vi "PV generator zen42 Laurent V3.vi"(8 "errin":errorcluster, 10 "network":path, 11 "path in":path) -> (0 "sortie d'erreur":errorcluster caption="errout", 2 "network out":path, 3 "tout bon":bool)   [LabVIEW 2017]
uses:
  <vilib>/Utility/config.llb/NI_LVConfig.lvlib
panel:
  out "Array 3":dbl[](array[numeric])
  out "nombre de remplacements":i32
  out "Chaîne":string
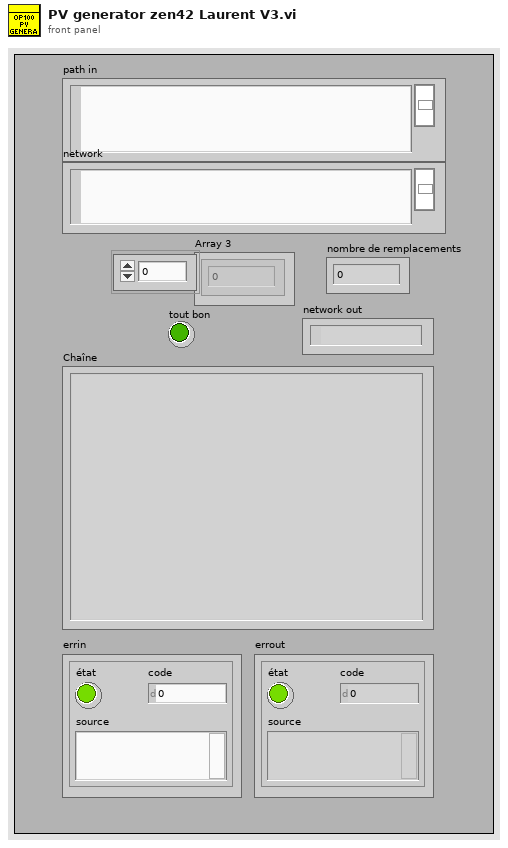
[diagram p1: front panel]
types:
  T1 = enum16{"open", "replace", "create", "open or create", "replace or create", "replace or create with confirmation"}
  T2 = typedef "NI_LVConfig.lvlib/Config Data RefNum.ctl" = refnum<k1>
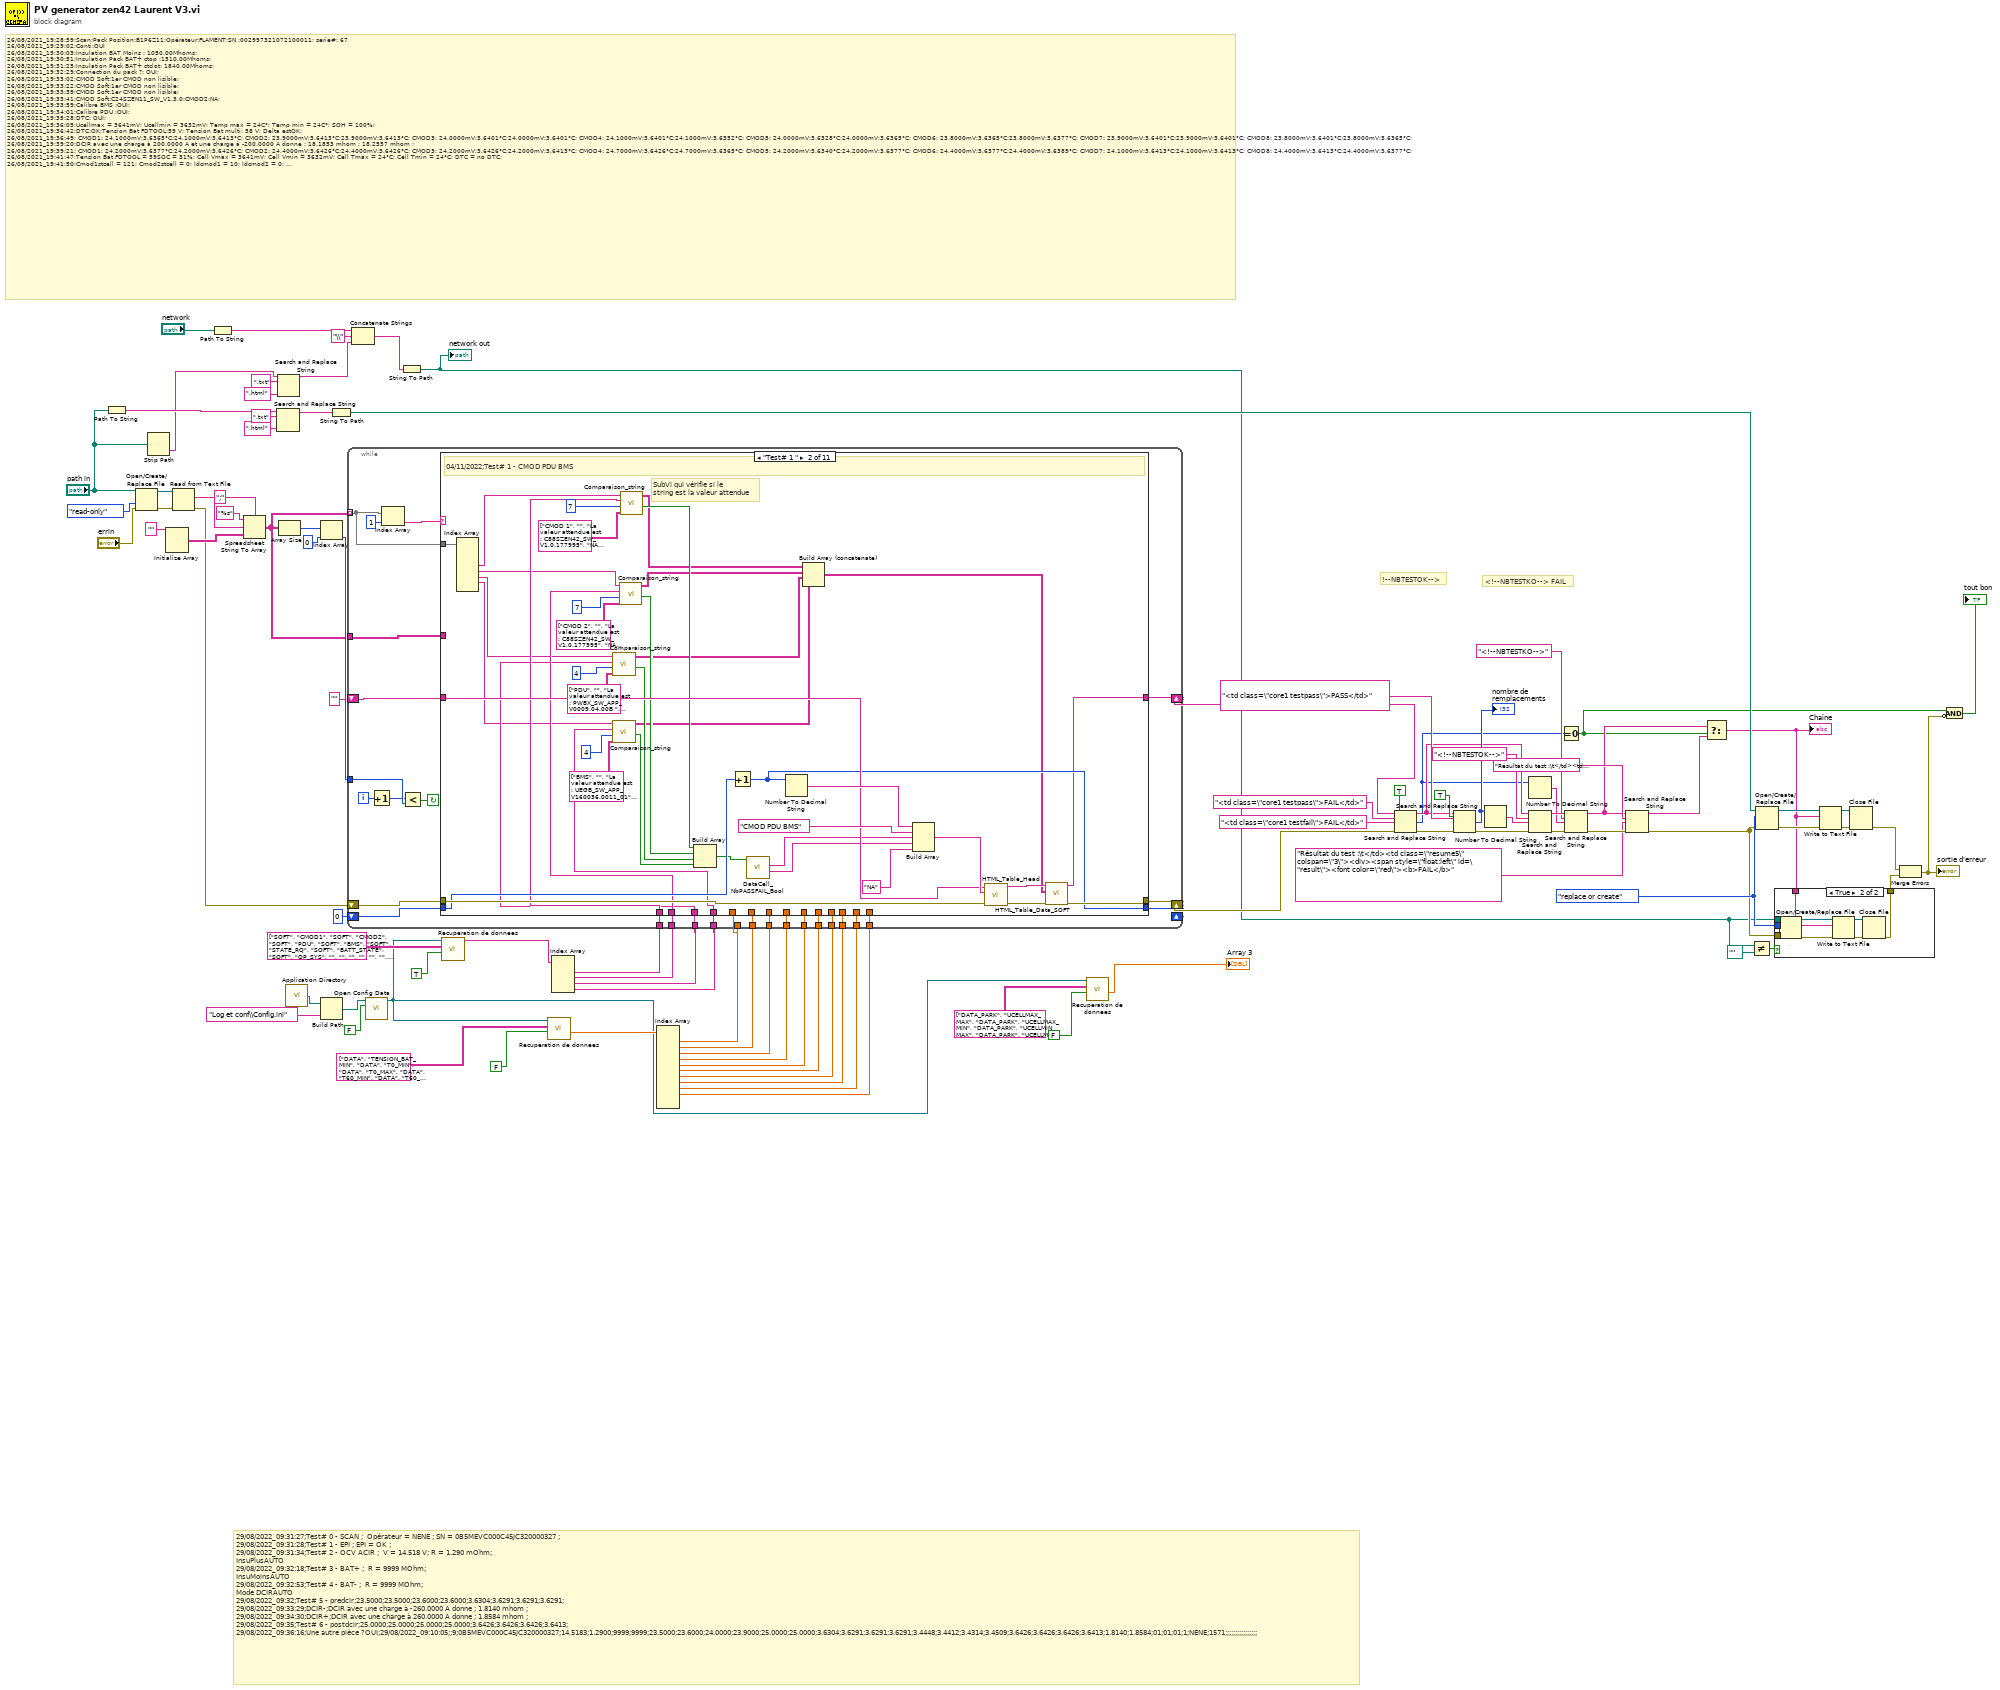
[diagram p0: block diagram]
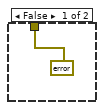
[diagram p2: hidden frame]
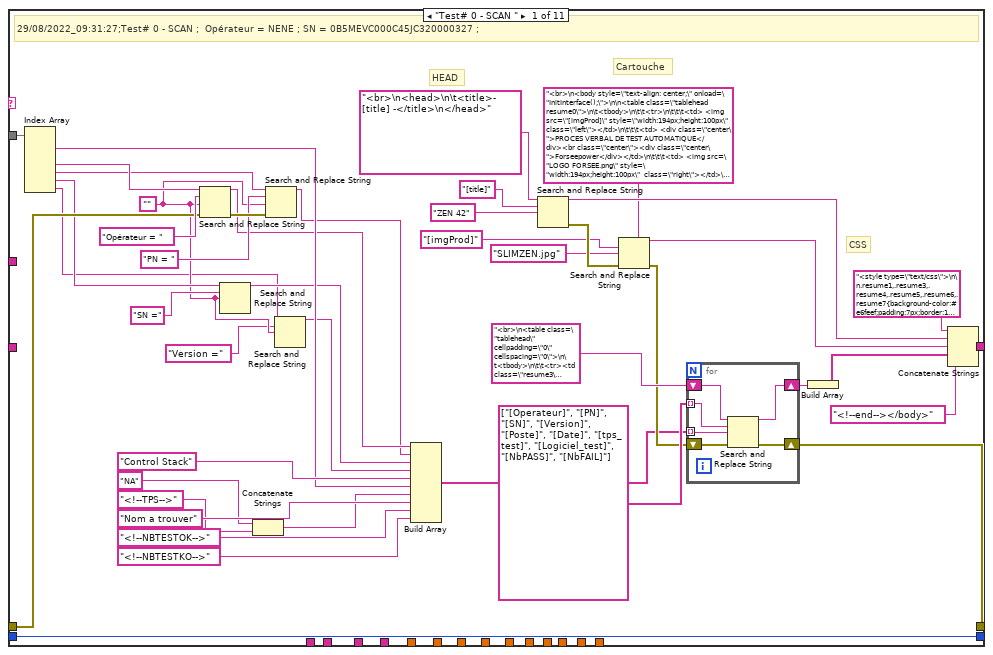
[diagram p3: hidden frame]
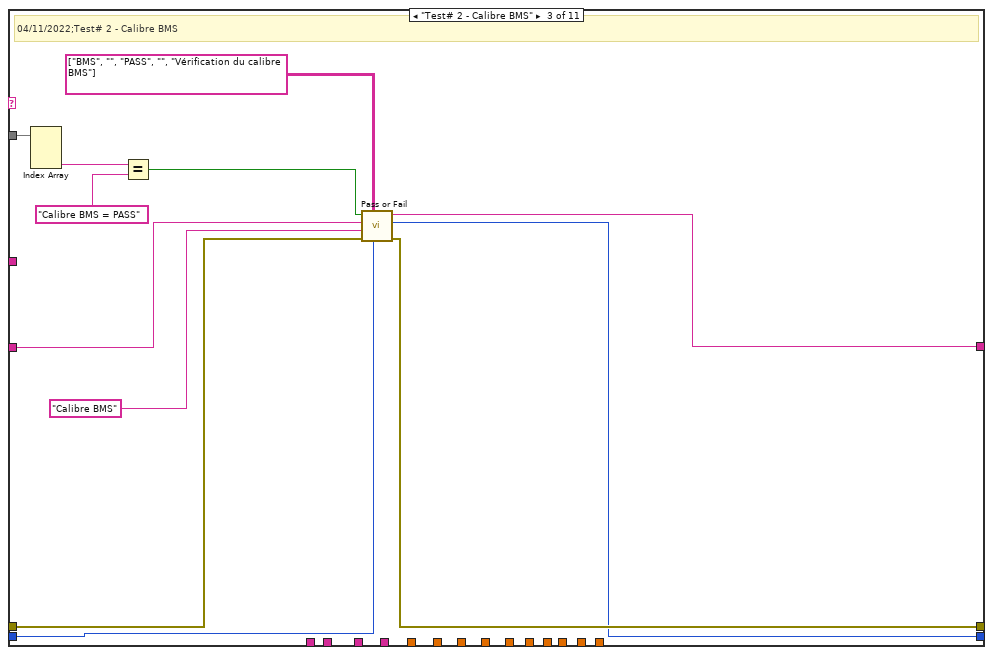
[diagram p4: hidden frame]
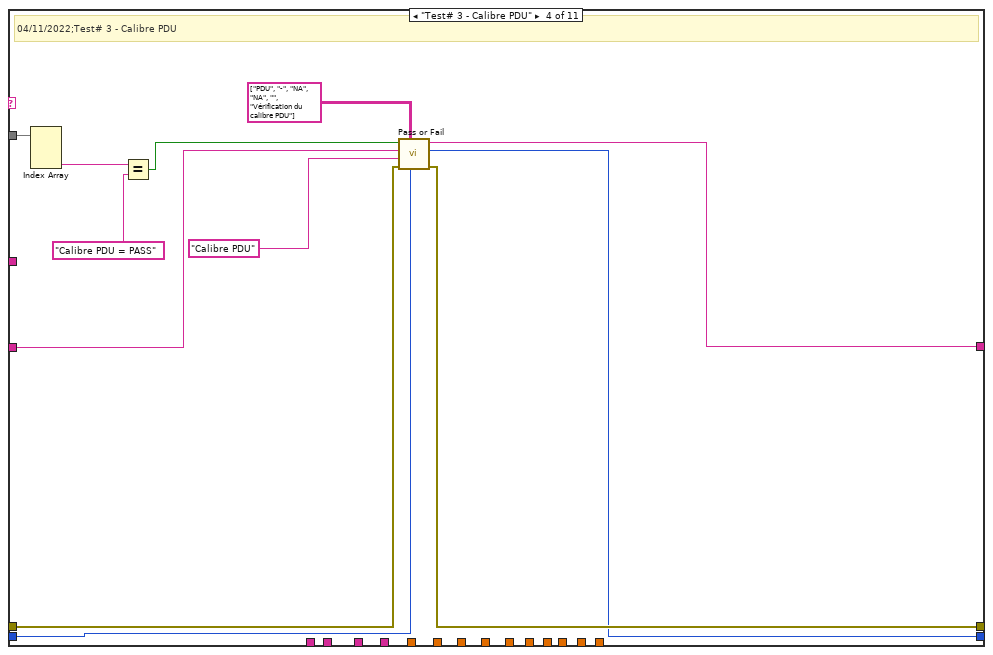
[diagram p5: hidden frame]
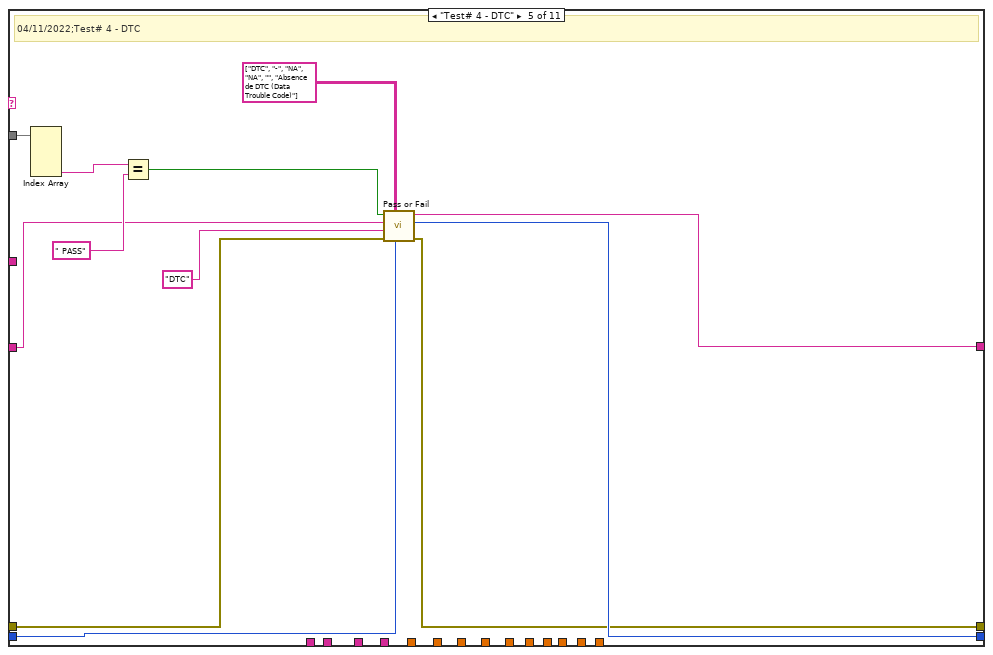
[diagram p6: hidden frame]
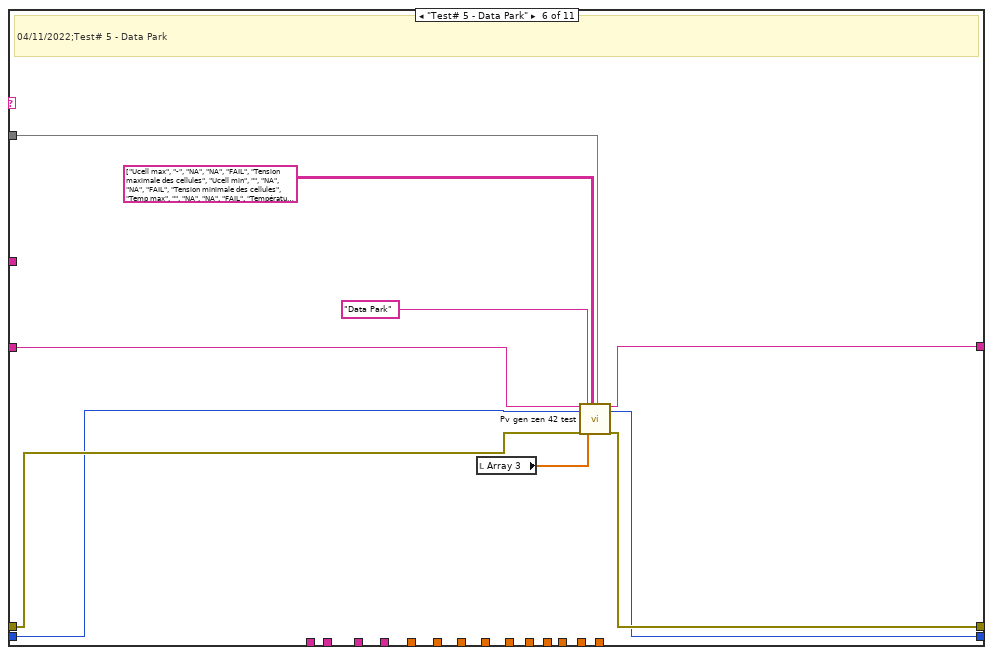
[diagram p7: hidden frame]
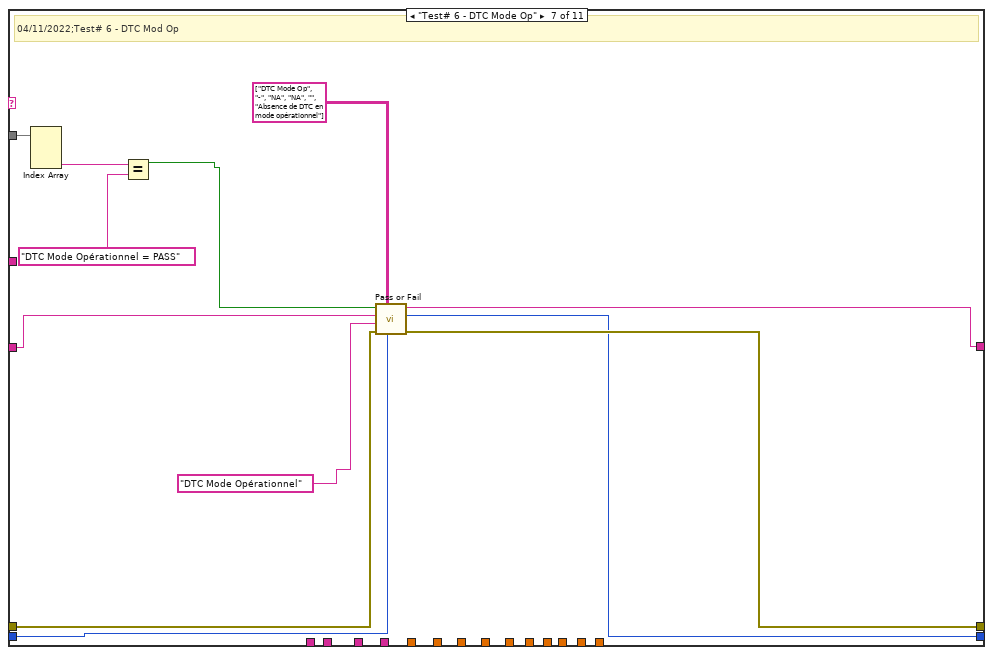
[diagram p8: hidden frame]
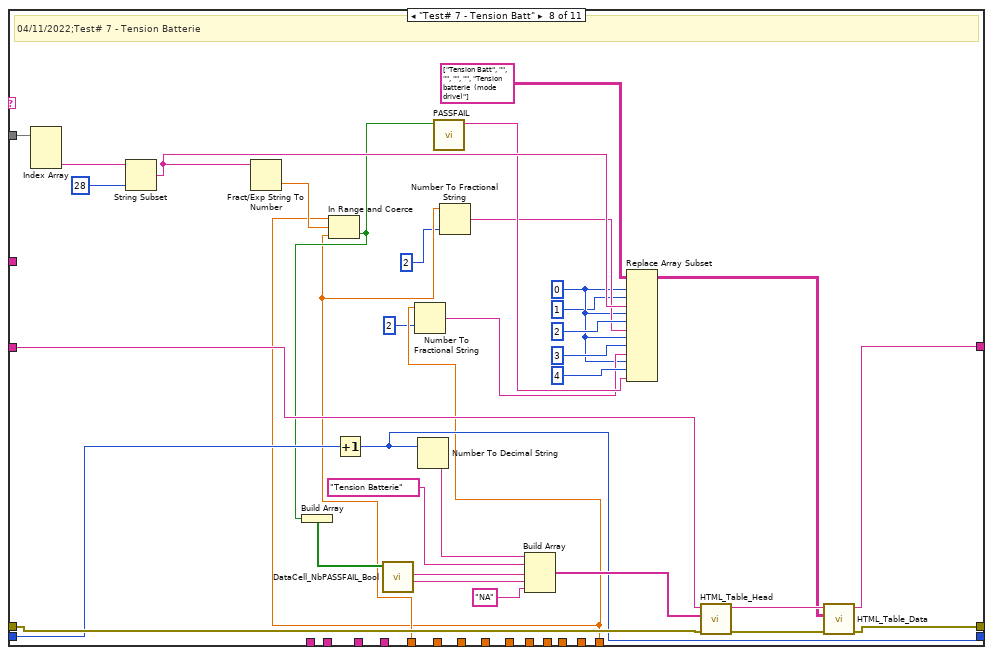
[diagram p9: hidden frame]
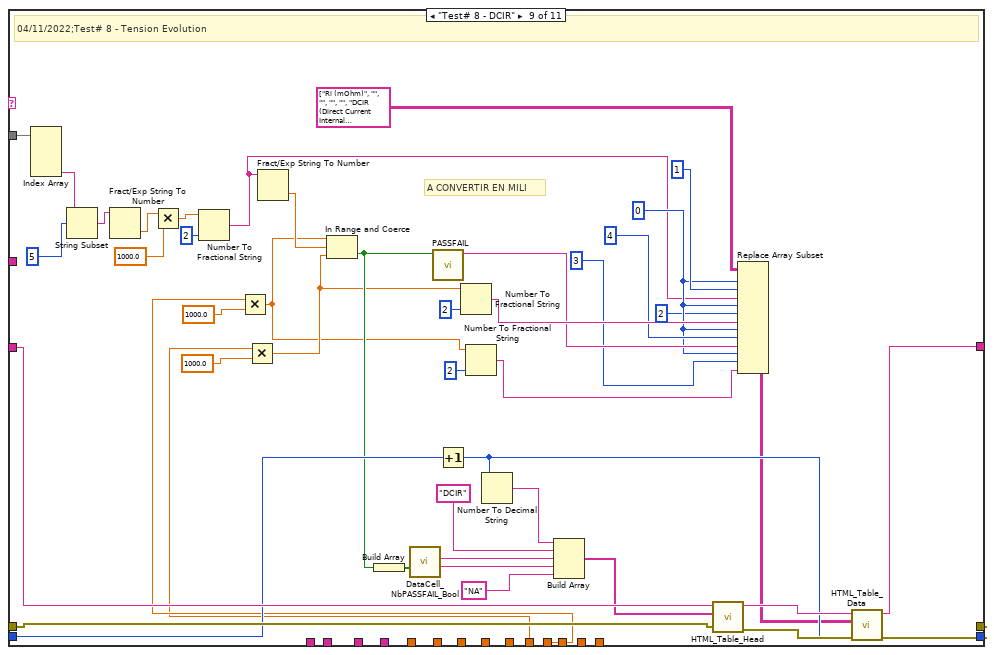
[diagram p10: hidden frame]
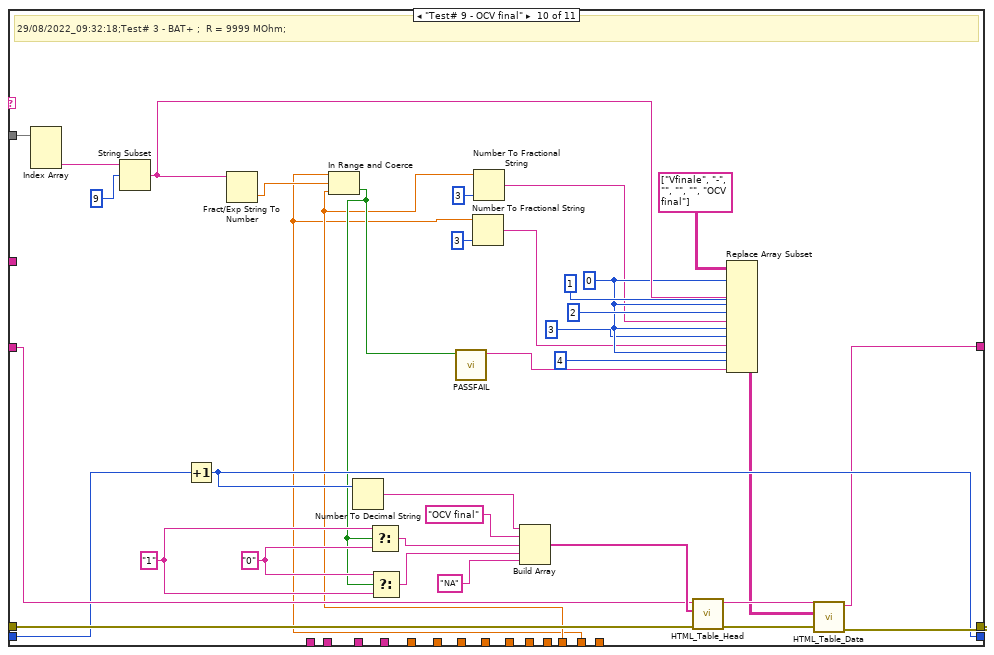
[diagram p11: hidden frame]
diagram:
  w54 = T1."replace or create" ("opération (0 : open)")
  # "29/08/2022_09:31:27;Test# 0 - SCAN ;  Opérateur = NENE ; SN = 0B5MEVC000C45JC320000327 ;\n29/08/2022_09:31:28;Test# 1 - EPI ; EPI = OK ;\n29/08/2022_09:31:34;Test# 2 - OCV ACIR ;  V = 14.518 V; R = 1.290 mOhm;\nInsuPlusAUTO\n29/08/2022_09:32:18;Test# 3 - BAT+ ;  R = 9999 MOhm;\nInsuMoinsAUTO\n29/08/2022_09:32:53;Test# 4 - BAT- ;  R = 9999 MOhm;\nMode DCIRAUTO\n29/08/2022_09:32;Test# 5 - predcir;23.5000;23.5000;23.6000;23.6000;3.6304;3.6291;3.6291;3.6291;\n29/08/2022_09:33:29;DCIR-;DCIR avec une charge à -260.0000 A donne ; 1.8140 mhom ; \n29/08/2022_09:34:30;DCIR+;DCIR avec une charge à 260.0000 A donne ; 1.8584 mhom ; \n29/08/2022_09:35;Test# 6 - postdcir;25.0000;25.0000;25.0000;25.0000;3.6426;3.6426;3.6426;3.6413;\n29/08/2022_09:36:16;Une autre pièce ?OUI;29/08/2022_09:10:05;;9;0B5MEVC000C45JC320000327;14.5183;1.2900;9999;9999;23.5000;23.6000;24.0000;23.9000;25.0000;25.0000;3.6304;3.6291;3.6291;3.6291;3.4448;3.4412;3.4314;3.4509;3.6426;3.6426;3.6426;3.6413;1.8140;1.8584;01;01;01;1;NENE;1571;;;;;;;;;;;;;;;;"
  # "<!--NBTESTKO--> FAIL"
  # "!--NBTESTOK-->"
  # "26/08/2021_19:28:59;Scan;Pack Position:B1P6Z11;Opérateur:FLAMENT;SN :002997321072100011; serie#: 67\n26/08/2021_19:29:02;Conti:OUI\n26/08/2021_19:30:03;Insulation BAT Moins : 1050.00Mhoms;\n26/08/2021_19:30:51;Insulation Pack BAT+ ctop :1510.00Mhoms;\n26/08/2021_19:31:25;Insulation Pack BAT+ ctclot: 1840.00Mhoms;\n26/08/2021_19:32:29;Connection du pack ?: OUI;\n26/08/2021_19:33:02;CMOD Soft:1er CMOD non lisible;\n26/08/2021_19:33:22;CMOD Soft:1er CMOD non lisible;\n26/08/2021_19:33:39;CMOD Soft:1er CMOD non lisible;\n26/08/2021_19:33:41;CMOD Soft:C24SZEN11_SW_V1.3.0;CMOD2:NA;\n26/08/2021_19:33:59;Calibre BMS :OUI;\n26/08/2021_19:34:01;Calibre PDU :OUI;\n26/08/2021_19:35:28;DTC: OUI;\n26/08/2021_19:36:05;Ucellmax = 3641mV; Ucellmin = 3632mV; Temp max = 24C°; Temp min = 24C°; SOH = 100%;\n26/08/2021_19:36:42;DTC:OK;Tension Bat FDTOOL:59 V; Tension Bat multi: 58 V; Delta estOK;\n26/08/2021_19:36:49; CMOD1: 24.1000mV;3.6365°C;24.1000mV;3.6413°C; CMOD2: 23.9000mV;3.6413°C;23.9000mV;3.6413°C; CMOD3: 24.0000mV;3.6401°C;24.0000mV;3.6401°C; CMOD4: 24.1000mV;3.6401°C;24.1000mV;3.6352°C; CMOD5: 24.0000mV;3.6328°C;24.0000mV;3.6365°C; CMOD6: 23.8000mV;3.6365°C;23.8000mV;3.6377°C; CMOD7: 23.9000mV;3.6401°C;23.9000mV;3.6401°C; CMOD8: 23.8000mV;3.6401°C;23.8000mV;3.6365°C;\n26/08/2021_19:39:20;DCIR avec une charge à 200.0000 A et une charge à -200.0000 A donne ; 18.1853 mhom ; 18.2557 mhom ; \n26/08/2021_19:39:21; CMOD1: 24.2000mV;3.6377°C;24.2000mV;3.6426°C; CMOD2: 24.4000mV;3.6426°C;24.4000mV;3.6426°C; CMOD3: 24.2000mV;3.6426°C;24.2000mV;3.6413°C; CMOD4: 24.7000mV;3.6426°C;24.7000mV;3.6365°C; CMOD5: 24.2000mV;3.6340°C;24.2000mV;3.6377°C; CMOD6: 24.4000mV;3.6377°C;24.4000mV;3.6389°C; CMOD7: 24.1000mV;3.6413°C;24.1000mV;3.6413°C; CMOD8: 24.4000mV;3.6413°C;24.4000mV;3.6377°C;\n26/08/2021_19:41:47;Tension Bat FDTOOL = 59SOC = 31%; Cell Vmax = 3641mV; Cell Vmin = 3632mV; Cell Tmax = 24°C; Cell Tmin = 24°C; DTC = no DTC;\n26/08/2021_19:41:50;Cmod1stcell = 121; Cmod2stcell = 0; Idcmod1 = 10; Idcmod2 = 0; ReId = KO;\n26/08/2021_19:42:38;Next ? PAS OK"
  n1 = Path To String(path="path in") -> (string=w76:string)
  n2 = Open/Create/Replace File(file path (use dialog)="path in", error in="errin", access (0:read/write)=enum16{"read/write", "read-only", "write-only"}."read-only" ("accès (0 : read/write)")) -> (refnum out=w77:refnum<file>, error out=w95:errorcluster)  [unwired: 3 in, 1 out]
  n3 = Strip Path(path="path in") -> (name=w34:string)  [unwired: 1 out]
  n4 = Initialize Array("") -> (w93:string[][])  [unwired: 2 in]
  n5 = Read from Text File(file (use dialog)=w77, error in=w95) -> (text=w91:string, error out=w82:errorcluster)  [unwired: 2 in, 2 out]
  n6 = Path To String(path="network") -> (string=w33:string)
  n7 = Spreadsheet String To Array(delimiter (Tab)=";" ("séparateur (Tabulation)"), format string="%s" ("chaîne de format"), spreadsheet string=w91, array type (2D Dbl)=w93) -> (array=w85:string[][])
  n8 = Search and Replace String(input string=w76, search string=".txt" ("chaîne recherchée"), replace string=".html" ("chaîne de remplacement (\"\")")) -> (result string=w73:string)  [unwired: 5 in, 3 out]
  n9 = Search and Replace String(input string=w34, search string=".txt" ("chaîne recherchée"), replace string=".html" ("chaîne de remplacement (\"\")")) -> (result string=w31:string)  [unwired: 5 in, 3 out]
  n10 = Array Size(array=w85) -> (size(s)=w89:i32[])
  n11 = call <vilib>:"Application Directory.vi"() -> ("Application Directory"=w9:path)
  n12 = Index Array(array=w89, index=0 ("indice")) -> (element=w87:i32)
  n13 = Build Path(base path=w9, name or relative path="Log et conf\\Config.ini") -> (appended path=w28:path)
  n14 = String To Path(string=w73) -> (path=w72:path)
  n15 = Concatenate Strings(w33, "\\" ("chaîne"), w31) -> (w30:string)
  n16 = call <vilib>:"Open Config Data.vi"("create file if necessary (T)"=FALSE, "configuration file path"=w28) -> ("refnum"=w3:T2)  [unwired: 7 in, 2 out]
  n17 = String To Path(string=w30) -> (path=w36:path)
  "network out" <- w36
  n18 = call "Recuperation de donnees.vi"("Est-ce un string?"=TRUE, "Array in"=string[][] [["SOFT", "CMOD1"], ["SOFT", "CMOD2"], ["SOFT", "PDU"], ["SOFT", "BMS"], ["SOFT", "STATE_RQ"], ["SOFT", "BATT_STATE"], ["SOFT", "OP_SYS"], ["", ""], ["", ""], ["", ""], ["", ""], ["", ""], ["", ""]], "Refnum in"=w3) -> ("String out"=w10:string[])  [unwired: 7 in, 1 out]
  n19 = call "Recuperation de donnees.vi"("Est-ce un string?"=FALSE, "Array in"=string[][] [["DATA", "TENSION_BAT_MIN"], ["DATA", "T0_MIN"], ["DATA", "T0_MAX"], ["DATA", "T60_MIN"], ["DATA", "T60_MAX"], ["DATA", "RI_MIN"], ["DATA", "RI_MAX"], ["DATA", "VF_MIN"], ["DATA", "VF_MAX"], ["DATA", "TENSION_BAT_MAX"], ["", ""], ["", ""], ["", ""]], "Refnum in"=w3) -> ("Array"=w5:dbl[])  [unwired: 7 in, 1 out]
  n20 = Index Array(array=w10) -> (element #1=w25:string, element #2=w24:string, element #3=w23:string, element #4=w22:string)  [unwired: 4 in]
  n21 = Index Array(array=w5) -> (element #1=w21:dbl, element #2=w19:dbl, element #3=w18:dbl, element #4=w17:dbl, element #5=w16:dbl, element #6=w15:dbl, element #7=w14:dbl, element #8=w13:dbl, element #9=w12:dbl, element #10=w11:dbl)  [unwired: 12 in, 2 out]
  n22 = while {
    tunnel: w87 -> [w123]
    tunnel: w85 -> [w120] mode=indexing
    shift-right: [w119] -> w69
    shift-left: w82 -> [w118]
    shift-right: [w112] -> w71
    shift-left: "" -> [w117]
    shift-right: [w115] -> _
    shift-left: 0 -> [w116]
    tunnel: w85 -> [w114]
    tunnel: w25 -> [w110]
    tunnel: w24 -> [w109]
    tunnel: w23 -> [w107]
    tunnel: w22 -> [w108]
    tunnel: w21 -> [w106]
    tunnel: w19 -> [w105]
    tunnel: w18 -> [w104]
    tunnel: w17 -> [w103]
    tunnel: w16 -> [w102]
    tunnel: w15 -> [w101]
    tunnel: w14 -> [w100]
    tunnel: w13 -> [w99]
    tunnel: w12 -> [w98]
    tunnel: w11 -> [w97]
    i -> [w124]
    stop <- w122 continue-if-true
    n23 = Increment(x=w124) -> (x+1=w113:i32)
    n24 = Index Array(array=w120, index=1 ("indice")) -> (element=w111:string)
    n25 = Less?(x=w113, y=w123) -> (x < y?=w122:bool)
    n26 = case shown="\"Test# 1 \"" w111 {
      tunnel: w118 -> [w166 w208 w224 w228 w243 w261 w266 w300 w345 w375 w391]
      tunnel: w120 -> [w168 w209 w225 w239 w251 w255 w273 w301 w346 w376 _]
      tunnel: [w138 w207 w223 w234 w244 w260 w265 w299 w344 w374 w391] -> w119
      tunnel: w117 -> [_ w206 w222 w232 w242 w253 w268 w298 w343 w373 w389]
      tunnel: w116 -> [w137 w205 w221 w229 w245 w254 w262 w297 w342 w372 w390]
      tunnel: [w137 w204 w220 w230 w246 w259 w263 w296 w341 w371 w390] -> w115
      tunnel: w114 -> [_ _ _ _ _ _ _ _ _ _ _]
      tunnel: [w136 w203 w219 w233 w240 w258 w264 w295 w309 w370 w389] -> w112
      tunnel: w110 -> [_ w201 _ _ _ _ _ _ _ _ _]
      tunnel: w109 -> [_ w193 _ _ _ _ _ _ _ _ _]
      tunnel: w108 -> [_ w186 _ _ _ _ _ _ _ _ _]
      tunnel: w107 -> [_ w190 _ _ _ _ _ _ _ _ _]
      tunnel: w106 -> [_ _ _ _ _ _ _ w283 _ _ _]
      tunnel: w105 -> [_ _ _ _ _ _ _ _ _ _ _]
      tunnel: w104 -> [_ _ _ _ _ _ _ _ _ _ _]
      tunnel: w103 -> [_ _ _ _ _ _ _ _ _ _ _]
      tunnel: w102 -> [_ _ _ _ _ _ _ _ _ _ _]
      tunnel: w101 -> [_ _ _ _ _ _ _ _ w312 _ _]
      tunnel: w100 -> [_ _ _ _ _ _ _ _ w313 _ _]
      tunnel: w99 -> [_ _ _ _ _ _ _ _ _ w354 _]
      tunnel: w98 -> [_ _ _ _ _ _ _ _ _ w353 _]
      tunnel: w97 -> [_ _ _ _ _ _ _ w280 _ _ _]
      frame "Test# 0 - SCAN " {
        w127 = ""
        # "Cartouche"
        # "HEAD"
        # "CSS"
        # "29/08/2022_09:31:27;Test# 0 - SCAN ;  Opérateur = NENE ; SN = 0B5MEVC000C45JC320000327 ;"
        n27 = Index Array(array=w168) -> (element #1=w139:string, element #3=w135:string, element #4=w134:string, element #5=w131:string, element #6=w126:string)  [unwired: 6 in, 1 out]
        n28 = Search and Replace String(input string=w135, search string="Opérateur = " ("chaîne recherchée"), replace string=w127, error in=w166) -> (result string=w133:string, error out=w165:errorcluster)  [unwired: 4 in, 2 out]
        n29 = Search and Replace String(input string=w131, search string="SN =" ("chaîne recherchée"), replace string=w127) -> (result string=w129:string)  [unwired: 5 in, 3 out]
        n30 = Concatenate Strings("NA" ("chaîne"), "<!--TPS-->" ("chaîne")) -> (w144:string)
        n31 = Search and Replace String(input string=w134, search string="PN = ", replace string=w127, error in=w165) -> (result string=w132:string)  [unwired: 4 in, 3 out]
        n32 = Search and Replace String(input string=w126, search string="Version =" ("chaîne recherchée"), replace string=w127) -> (result string=w128:string)  [unwired: 5 in, 3 out]
        n33 = Build Array(w133, w132, w129, w128, "Control Stack" ("chaîne"), w139, w144, "Nom a trouver" ("chaîne"), "<!--NBTESTOK-->" ("chaîne"), "<!--NBTESTKO-->" ("chaîne")) -> (w140:string[])
        n34 = Search and Replace String(input string="<br>\n<head>\n\t<title>- [title] -</title>\n</head>", search string="[title]" ("chaîne recherchée"), replace string="ZEN 42" ("Title")) -> (result string=w160:string, error out=w159:errorcluster)  [unwired: 5 in, 2 out]
        n35 = Search and Replace String(input string="<br>\n<body style=\"text-align: center;\" onload=\"InitInterface();\">\n\n<table class=\"tablehead resume0\">\n\t<tbody>\n\t\t<tr>\n\t\t\t<td> <img src=\"[imgProd]\" style=\"width:194px;height:100px\" class=\"left\"></td>\n\t\t\t<td> <div class=\"center\">PROCES VERBAL DE TEST AUTOMATIQUE</div><br class=\"center\"><div class=\"center\">Forseepower</div></td>\n\t\t\t<td> <img src=\"LOGO FORSEE.png\" style=\"width:194px;height:100px\"  class=\"right\"></td>\n\t\t</tr>\n\t</tbody>\n</table>", search string="[imgProd]", replace string="SLIMZEN.jpg" ("imgProd"), error in=w159) -> (result string=w156:string, error out=w153:errorcluster)  [unwired: 4 in, 2 out]
        n36 = for {
          shift-right: [w173] -> w152
          shift-left: "<br>\n<table class=\"tablehead\" cellpadding=\"0\" cellspacing=\"0\">\n\t<tbody>\n\t\t<tr><td class=\"resume3\">Opérateur :\t</td><td class=\"resume5\" colspan=\"3\">[Operateur]</td></tr>\n\t\t<tr><td class=\"resume3\">PN : </td><td class=\"resume5\" colspan=\"3\">[PN]</td></tr>\n\t\t<tr><td class=\"resume3\">SN : </td><td class=\"resume5\" colspan=\"3\">[SN]</td></tr>\n\t\t<tr><td class=\"resume3\">Version : </td><td class=\"resume5\" colspan=\"3\">[Version]</td></tr>\n\t\t<tr><td class=\"resume3\">Poste : </td><td class=\"resume5\" colspan=\"3\">[Poste]</td></tr>\t\t\n\t\t<tr><td class=\"resume3\">Date du test : </td><td class=\"resume5\" colspan=\"3\">[Date]</td></tr>\n\t\t<tr><td class=\"resume3\">Temps de test : </td><td class=\"resume5\" colspan=\"3\">[tps_test]</td></tr>\n\t\t<tr><td class=\"resume3\">Logiciel de test :\t</td><td class=\"resume5\" colspan=\"3\">[Logiciel_test]</td></tr>\n\t\t<tr><td class=\"resume3\">Résultat du test :\t</td><td class=\"resume5\" colspan=\"3\"><div><span style=\"float:left\" id=\"result\"><font color=\"green\"><b>PASS</b></font><b> ( <font color=\"green\">[NbPASS] PASS</font> / <font color=\"red\">[NbFAIL] FAIL</font> )</b></span></div></td></tr>\n\t</tbody>\n</table>" -> [w174]
          tunnel: string[] ["[Operateur]", "[PN]", "[SN]", "[Version]", "[Poste]", "[Date]", "[tps_test]", "[Logiciel_test]", "[NbPASS]", "[NbFAIL]"] -> [w170] mode=indexing
          tunnel: w140 -> [w169] mode=indexing
          shift-right: [w171] -> w138
          shift-left: w153 -> [w172]
          n37 = Search and Replace String(input string=w174, search string=w170, replace string=w169, error in=w172) -> (result string=w173:string, error out=w171:errorcluster)  [unwired: 4 in, 2 out]
        }
        n38 = Build Array(w152) -> (w151:string[])
        n39 = Concatenate Strings("<style type=\"text/css\">\n\n.resume1,.resume3,.resume4,.resume5,.resume6,.resume7{background-color:#e6feef;padding:7px;border:1px solid black;}\n.resume0{border:1px solid black;background-color:#e6feef;font-weight: bold;padding:0px;text-align: center;}\n.resume1{width:350px;text-align:right;font-weight:bold;}\n.resume3{width:350px;text-align:right;border-top:0px solid black;font-weight:bold;}\n.resume4{border-left:0px solid black;width:290px;}\n.resume5{width:290px;border-left:0px solid black;border-top:0px solid black;}\n.resume6{border-left:0px solid black;width:60px;}\n.resume7{border-left:0px solid black;border-top:0px solid black;width:60px;}\n.title1{text-align: left;background-color:#e6f4fe;padding:10px;border:1px solid #101010;}\n.title2{width: 30px;text-align: center;background-color:#e6f4fe;padding:1px;border:1px solid #101010;border-left:0px solid black;font-weight: bold;}\n.title2 a:link{text-decoration:none;}\n.entete0,.entete1,.entete2,.time2{text-align: center;background-color:#feeec9;padding:7px;border:1px solid black;font-weight: bold;}\n.entete0{width:45px;border-right:0px solid black;}\n.entete1{width:505px;}\n.entete2{width:95px;border-right:0px solid black;}\n.time2{border-left:0px solid black;width:145px;font-size:11px;}\n.core0,.core1,.core2,.core3,.core4,.time{text-align: center;background-color:#fafed3;padding:7px;border:1px solid black;}\n.core0, .core1,.core3,.core4{width:95px;border-top:0px solid black;border-right:0px solid black;}\n.core0{width:45px;}\n.core2{border-top:0px solid black;width:505px;}\n.core3{width:200px;}\n.core4{width:300px;}\n.time{width:145px;border-top:0px solid black;border-left:0px solid black;font-size:11px;}\n.false .core0,.false .core1,.false .core2,.false .core3,.false .core4,.false .time{background-color:#f4f4f4;}\n.false .entete0,.false .entete1,.false .entete2,.false .time2{background-color:#dadada;}\n.false .title1,.false .title2,.false .resultentete .testpass,.false .resultentete .testfail,.false .resultentete .testtime{background-color:#c5cac9;color: blue;}\n.false .title2 a:link{text-decoration:none;color: blue;}\n.comment1,.comment2,.time3{width: 890px;background-color:#e9e8e9;padding:7px;border:1px solid black;border-top:0px solid black;text-align:left;}\n.comment2{border-right:0px solid black;width: 45px;text-align: center;}\n.time3{width: 145px;border-left:0px solid black;font-size:11px;}\n.fixe1{background: -moz-linear-gradient(center top , #101010 10%, #555555 80%) repeat scroll 0 0 transparent;background: -webkit-gradient(linear, left top, left bottom, from(#101010), to(#555555));border:2px solid orange;position : fixed;margin-top:20px;display:none;overflow-y:scroll;max-height:350px;text-shadow: 0px 0px 0 #333333;text-align:left;font-size:10px;padding:10px;margin-left:-162px;border-radius: 15px 15px 15px 15px;}\n.menufixe, .menufixelock{background: -moz-linear-gradient(center top , #101010 80%, transparent 20%) repeat scroll 0 0 transparent;background: -webkit-gradient(linear, left top, left bottom, from(#101010), color-stop(0.65, #101010), to(transparent)) repeat scroll 0 0 transparent;margin: -52px 0px 0px -9px;width:100%;position:fixed;height:55px;-moz-transition: margin 1s;-webkit-transition: margin 1s;}\n.menufixelock, .menufixe:hover{margin: -9px 0px 0px -9px;}\n.lockmenu, .separation,.separationmenu{text-align:center;background: -moz-linear-gradient(center top , #555555 10%, #111111 80%) repeat scroll 0 0 transparent;background: -webkit-gradient(linear, left top, left bottom, from(#555555), to(#111111));border: 1px solid white;border-radius: 10px 10px 10px 10px;box-shadow: 0 -1px 1px #555555 inset;color: #999999;font-weight: bold;width: 100px;padding: 2px;text-decoration: none;}\n.tablehead{width: 1000px;font-family: Verdana;font-size: 12px;margin-left: auto;margin-right: auto;}\n.tablenull{font-family: Verdana;font-size: 11px;margin-left: auto;margin-right: auto;}\n.separationmenu:hover div{display: inline;}\n.lockmenu:hover, .separation:hover,.separationmenu:hover{border: 1px solid orange;cursor:pointer;}\n.lockmenu:hover{border: 1px solid red;cursor:pointer;}\n.separationright{padding:10px;}\ndiv a:link{text-decoration:none;color:#cbcbcb;}\ndiv a:hover{text-decoration:underline;color:#cbcbcb;}\nspan a:link{text-decoration:none;color:#cbcbcb;}\nspan a:hover{text-decoration:none;color:#cbcbcb;}\n.false{color: blue;}\n.testpass{color: green;font-weight: bold;}\n.testfail{color: red;font-weight: bold;}\n.testtime{color: blue;font-weight: bold;}\n.resultentete{font-weight: bold;font-size: 11px;min-width: 200px;text-align:right;}\n.infohard{border: 1px solid black;background-color: white;text-align: center;width: 16px;height: 16px;border-radius: 5px;font-weight: bold;box-shadow: 0 -1px 2px #555555 inset;}\n.infohard:hover{background-color:#feeec9;cursor:pointer;}\n.footerhard{padding-top:30px;}\n.confighard{font-size:10px;width:110px;}\n.circlemain{margin-left:auto;margin-right:auto;}\n.circletext,.circleform{padding-top: 3px;text-align:center;font-size: 10px;width:200px;}\n.circleform{padding-bottom: 3px;padding-top: 1px;}\n.circle{border: 1px solid black;border-collapse: collapse;border-radius: 15px;box-shadow: 1px 1px 0 #505050;height: 15px;width: 15px;display:inline-block;}\n.bookmarkon, .bookmarkoff{background-color: yellow;border: 1px solid black;border-collapse: collapse;border-radius: 10px 10px 10px 10px;box-shadow: 1px 1px 0 #505050;height: 12px;width: 12px;position: absolute;margin-left:22px;cursor: help;}\n.bookmarkoff{background-color: transparent;border: 1px solid #CECECE;box-shadow: none;cursor: copy;}\n.false .bookmarkoff{background-color: transparent;border: 1px solid #E6E1E1;box-shadow: none;cursor: copy;}\n.bookmarkmaster{height: 15px;margin-right: 12px;width: 60px;}\n.bookmarkmaster:hover .bookmarkprev,.bookmarkmaster:hover .bookmarksuiv{display:block;}\n.bookmarkprev, .bookmarksuiv {cursor: pointer;font-size: 25px;font-weight: bold;margin-top: -10px;position: absolute;display:none;}\n.bookmarkprev{margin-left: 2px;}\n.bookmarksuiv{margin-left: 43px;}\n.plus, .moins{background-color: #F4F4F4;border: 1px solid #848484;border-radius: 20px;color: #848484;font-family: arial;font-size: 16px;font-weight: bold;height: 20px;margin-left: 4px;text-align: center;width: 20px;}\n.moins{font-size: 15px;}\n.plus:hover, .moins:hover{background-color: #DADADA;border: 1px solid black;color: black;cursor:pointer;}\n.backtothetop {position: fixed; right: 50%; margin-right: -555px; bottom: 10px; font-size: 35px; font-weight: bold; border: 1px solid #7D7B91; width: 40px; height: 40px; line-height:52px; text-align: center;border-radius: 8px; opacity: 0.25; background-color: #F5F5F5; color:#7D7B91;}\n.backtothetop:hover {opacity: 1; cursor:pointer;}\n.libversion {font-size: 8px;font-weight: normal;padding-right: 10px;text-align: right;}\n.lockmenu {width: 18px;font-size: 12px;}\n.left {display: block; margin-left: 1px;margin-right: auto;}\n.right {display: block; margin-right: 1px;margin-left: auto;}\n.center {display: block; margin-left: auto;margin-right: auto;}\n\n</style>", w160, w156, w151, "<!--end--></body>") -> (w136:string)
      }
      frame "Test# 1 " {
        # "SubVi qui vérifie si le \nstring est la valeur attendue"
        # "04/11/2022;Test# 1 - CMOD PDU BMS"
        n40 = Index Array(array=w209) -> (element #3=w202:string, element #4=w195:string, element #5=w192:string, element #6=w188:string)  [unwired: 7 in, 3 out]
        n41 = call "Comparaison_string.vi"("Ligne en cours"=string[][] [["PDU", "", "La valeur attendue est : PWBX_SW_APP_V0009.04.00B ", "NA", "", ""]] ("Tableau"), "offset lecture valeur"=4 ("offset (0)"), "valeur attendue"=w190, "Valeur lue"=w192) -> ("PASS / FAIL"=w189:bool, "output array"=w177:string[][])  [unwired: 6 in]
        n42 = call "Comparaison_string.vi"("Ligne en cours"=string[][] [["BMS", "", "La valeur attendue est : UEGB_SW_APP_V160036.0011_01", "NA", "", ""]] ("Tableau"), "offset lecture valeur"=4 ("offset (0)"), "valeur attendue"=w186, "Valeur lue"=w188) -> ("PASS / FAIL"=w185:bool, "output array"=w178:string[][])  [unwired: 6 in]
        n43 = call "Comparaison_string.vi"("Ligne en cours"=string[][] [["CMOD 2", "", "La valeur attendue est : C88SZEN42_SW_V1.0.177995", "NA", "", ""]] ("Tableau"), "offset lecture valeur"=7 ("offset (0)"), "valeur attendue"=w193, "Valeur lue"=w195) -> ("PASS / FAIL"=w184:bool, "output array"=w176:string[][])  [unwired: 6 in]
        n44 = call "Comparaison_string.vi"("Ligne en cours"=string[][] [["CMOD 1", "", "La valeur attendue est : C88SZEN42_SW_V1.0.177995", "NA", "", ""]] ("Tableau"), "offset lecture valeur"=7 ("offset (0)"), "valeur attendue"=w201, "Valeur lue"=w202) -> ("PASS / FAIL"=w200:bool, "output array"=w175:string[][])  [unwired: 6 in]
        n45 = Build Array(w200, w184, w189, w185) -> (w199:bool[])
        n46 = Increment(x=w205) -> (x+1=w204:i32)
        n47 = call "DataCell_NbPASSFAIL_Bool.vi"("Tableau en entrée"=w199) -> ("Chaîne"=w197:string, "Chaîne 2"=w198:string)  [unwired: 8 in, 1 out]
        n48 = Number To Decimal String(number=w204) -> (decimal integer string=w212:string)  [unwired: 1 in]
        n49 = Build Array (concatenate)(w175, w176, w177, w178) -> (w183:string[][])
        n50 = Build Array(w212, "CMOD PDU BMS" ("élément"), w198, w197, "NA" ("élément")) -> (w215:string[])
        n51 = call "HTML_Table_Head.vi"("entrée d'erreur (pas d'erreur)"=w208, "Tableau"=w215, "chaîne en entrée"=w206) -> ("sortie d'erreur"=w214:errorcluster, "result string"=w213:string)  [unwired: 7 in]
        n52 = call "HTML_Table_Data_SOFT.vi"("entrée d'erreur (pas d'erreur)"=w214, "Tableau"=w183, "chaîne en entrée"=w213) -> ("sortie d'erreur"=w207:errorcluster, "result string"=w203:string)  [unwired: 7 in]
      }
      frame "Test# 2 - Calibre BMS" {
        # "04/11/2022;Test# 2 - Calibre BMS"
        n53 = Index Array(array=w225) -> (element #3=w217:string)  [unwired: 3 in, 2 out]
        n54 = Equal?(x=w217, y="Calibre BMS = PASS") -> (x = y?=w216:bool)
        n55 = call "Pass or Fail.vi"("Numeric in"=w221, "Ligne à modifier"=string[][] [["BMS", "", "PASS", "", "Vérification du calibre BMS"]] ("Tableau"), "error in (no error)"=w224, "Nom test"="Calibre BMS" ("élément"), "String"=w222, "Boolean"=w216) -> ("error out"=w223:errorcluster, "Numeric out"=w220:i32, "tableau sortie"=w219:string)  [unwired: 3 in]
      }
      frame "Test# 3 - Calibre PDU" {
        # "04/11/2022;Test# 3 - Calibre PDU"
        n56 = Index Array(array=w239) -> (element #3=w237:string)  [unwired: 3 in, 2 out]
        n57 = Equal?(x=w237, y="Calibre PDU = PASS") -> (x = y?=w235:bool)
        n58 = call "Pass or Fail.vi"("Numeric in"=w229, "Ligne à modifier"=string[][] [["PDU", "-", "NA", "NA", "", "Vérification du calibre PDU"]] ("Tableau"), "error in (no error)"=w228, "Nom test"="Calibre PDU" ("élément"), "String"=w232, "Boolean"=w235) -> ("error out"=w234:errorcluster, "Numeric out"=w230:i32, "tableau sortie"=w233:string)  [unwired: 3 in]
      }
      frame "Test# 4 - DTC" {
        # "04/11/2022;Test# 4 - DTC"
        n59 = Index Array(array=w251) -> (element #4=w249:string)  [unwired: 4 in, 3 out]
        n60 = Equal?(x=w249, y=" PASS") -> (x = y?=w248:bool)
        n61 = call "Pass or Fail.vi"("Numeric in"=w245, "Ligne à modifier"=string[][] [["DTC", "-", "NA", "NA", "", "Absence de DTC (Data Trouble Code)"]] ("Tableau"), "error in (no error)"=w243, "Nom test"="DTC" ("élément"), "String"=w242, "Boolean"=w248) -> ("error out"=w244:errorcluster, "Numeric out"=w246:i32, "tableau sortie"=w240:string)  [unwired: 3 in]
      }
      frame "Test# 5 - Data Park" {
        # "04/11/2022;Test# 5 - Data Park"
        n62 = local read "Array 3"() -> (w252:dbl[])
        n63 = call "Pv gen zen 42 test.vi"("FluxStrIn"=w253, "Numin"=w254, "errin"=w261, "testlabel"="Data Park" ("élément"), "Data limit"=w252, "tab ref"=string[][] [["Ucell max", "-", "NA", "NA", "FAIL", "Tension maximale des cellules"], ["Ucell min", "", "NA", "NA", "FAIL", "Tension minimale des cellules"], ["Temp max", "", "NA", "NA", "FAIL", "Température maximale des cellules"], ["Temp min", "", "NA", "NA", "FAIL", "Température minimale des cellules"], ["SOH", "", "NA", "NA", "FAIL", "State Of Heal"], ["SOC", "", "NA", "NA", "FAIL", "State Of Charge"], ["Vbatt", "", "NA", "NA", "FAIL", "Tension de la batterie"], ["Ibatt", "", "NA", "NA", "FAIL", "Courant de la batterie"]] ("Tableau"), "ligne à traiter"=w255) -> ("result string"=w258:string, "Numout"=w259:i32, "errout"=w260:errorcluster)  [unwired: 10 in]
      }
      frame "Test# 6 - DTC Mode Op" {
        # "04/11/2022;Test# 6 - DTC Mod Op"
        n64 = Index Array(array=w273) -> (element #3=w271:string)  [unwired: 3 in, 2 out]
        n65 = Equal?(x=w271, y="DTC Mode Opérationnel = PASS") -> (x = y?=w269:bool)
        n66 = call "Pass or Fail.vi"("Numeric in"=w262, "Ligne à modifier"=string[][] [["DTC Mode Op", "-", "NA", "NA", "", "Absence de DTC en mode opérationnel"]] ("Tableau"), "error in (no error)"=w266, "Nom test"="DTC Mode Opérationnel" ("élément"), "String"=w268, "Boolean"=w269) -> ("error out"=w265:errorcluster, "Numeric out"=w263:i32, "tableau sortie"=w264:string)  [unwired: 3 in]
      }
      frame "Test# 7 - Tension Batt" {
        w277 = 0 ("index (row)")
        # "04/11/2022;Test# 7 - Tension Batterie"
        n67 = Index Array(array=w301) -> (element #3=w293:string)  [unwired: 3 in, 2 out]
        n68 = String Subset(string=w293, offset (0)=28) -> (substring=w285:string)  [unwired: 1 in]
        n69 = Fract/Exp String To Number(string=w285) -> (number=w282:dbl)  [unwired: 3 in, 1 out]
        n70 = In Range and Coerce(upper limit=w280, x=w282, lower limit=w283) -> (In Range?=w284:bool)  [unwired: 1 out]
        n71 = Build Array(w284) -> (w291:bool[])
        n72 = Increment(x=w297) -> (x+1=w296:i32)
        n73 = call "DataCell_NbPASSFAIL_Bool.vi"("Tableau en entrée"=w291) -> ("Chaîne"=w289:string, "Chaîne 2"=w290:string)  [unwired: 8 in, 1 out]
        n74 = Number To Fractional String(number=w280, precision (6)=i16 2) -> (F-format string=w278:string)  [unwired: 2 in]
        n75 = Number To Decimal String(number=w296) -> (decimal integer string=w304:string)  [unwired: 1 in]
        n76 = call "PASSFAIL.vi"("E"=w284) -> ("S"=w281:string)  [unwired: 10 in]
        n77 = Number To Fractional String(number=w283, precision (6)=i16 2) -> (F-format string=w279:string)  [unwired: 2 in]
        n78 = Build Array(w304, "Tension Batterie" ("élément"), w290, w289, "NA" ("élément")) -> (w307:string[])
        n79 = Replace Array Subset(array=string[][] [["Tension Batt", "", "", "", "", "Tension batterie  (mode drive)"]] ("Tableau"), new element #1=w285, index (row) #1=w277, index (col) #1=1 ("disabled index (col)"), new element #2=w279, index (row) #2=w277, index (col) #2=2 ("disabled index (col)"), new element #3=w278, index (row) #3=w277, index (col) #3=3 ("disabled index (col)"), new element #4=w281, index (row) #4=w277, index (col) #4=4 ("disabled index (col)")) -> (w294:string[][])
        n80 = call "HTML_Table_Head.vi"("entrée d'erreur (pas d'erreur)"=w300, "Tableau"=w307, "chaîne en entrée"=w298) -> ("sortie d'erreur"=w306:errorcluster, "result string"=w305:string)  [unwired: 7 in]
        n81 = call "HTML_Table_Data.vi"("entrée d'erreur (pas d'erreur)"=w306, "Tableau"=w294, "chaîne en entrée"=w305) -> ("sortie d'erreur"=w299:errorcluster, "result string"=w295:string)  [unwired: 7 in]
      }
      frame "Test# 8 - DCIR" {
        w327 = 0 ("disabled index (col)")
        # "A CONVERTIR EN MILI"
        # "04/11/2022;Test# 8 - Tension Evolution"
        n82 = Index Array(array=w346) -> (element #4=w333:string)  [unwired: 4 in, 3 out]
        n83 = String Subset(string=w333, offset (0)=5) -> (substring=w321:string)  [unwired: 1 in]
        n84 = Fract/Exp String To Number(string=w321) -> (number=w320:dbl)  [unwired: 3 in, 1 out]
        n85 = Multiply(x=w320, y=1000.0) -> (x*y=w318:dbl)
        n86 = Number To Fractional String(number=w318, precision (6)=i16 2) -> (F-format string=w317:string)  [unwired: 2 in]
        n87 = Multiply(x=w313, y=1000.0) -> (x*y=w310:dbl)
        n88 = Multiply(x=w312, y=1000.0) -> (x*y=w311:dbl)
        n89 = Fract/Exp String To Number(string=w317) -> (number=w335:dbl)  [unwired: 3 in, 1 out]
        n90 = In Range and Coerce(upper limit=w310, x=w335, lower limit=w311) -> (In Range?=w334:bool)  [unwired: 1 out]
        n91 = Build Array(w334) -> (w338:bool[])
        n92 = call "DataCell_NbPASSFAIL_Bool.vi"("Tableau en entrée"=w338) -> ("Chaîne"=w336:string, "Chaîne 2"=w337:string)  [unwired: 8 in, 1 out]
        n93 = call "PASSFAIL.vi"("E"=w334) -> ("S"=w328:string)  [unwired: 10 in]
        n94 = Increment(x=w342) -> (x+1=w341:i32)
        n95 = Number To Fractional String(number=w311, precision (6)=i16 2) -> (F-format string=w330:string)  [unwired: 2 in]
        n96 = Number To Fractional String(number=w310, precision (6)=i16 2) -> (F-format string=w325:string)  [unwired: 2 in]
        n97 = Number To Decimal String(number=w341) -> (decimal integer string=w349:string)  [unwired: 1 in]
        n98 = Build Array(w349, "DCIR" ("élément"), w337, w336, "NA" ("élément")) -> (w332:string[])
        n99 = call "HTML_Table_Head.vi"("entrée d'erreur (pas d'erreur)"=w345, "Tableau"=w332, "chaîne en entrée"=w343) -> ("sortie d'erreur"=w351:errorcluster, "result string"=w350:string)  [unwired: 7 in]
        n100 = Replace Array Subset(array=string[][] [["Ri (mOhm)", "", "", "", "", "DCIR (Direct Current Internal Resistance="]] ("Tableau"), new element #1=w317, index (row) #1=w327, index (col) #1=1 ("indice désactivé (col)"), new element #2=w330, index (row) #2=w327, index (col) #2=2 ("disabled index (col)"), new element #3=w328, index (row) #3=w327, index (col) #3=4 ("disabled index (col)"), new element #4=w325, index (row) #4=w327, index (col) #4=3 ("disabled index (col)")) -> (w340:string[][])
        n101 = call "HTML_Table_Data.vi"("entrée d'erreur (pas d'erreur)"=w351, "Tableau"=w340, "chaîne en entrée"=w350) -> ("sortie d'erreur"=w344:errorcluster, "result string"=w309:string)  [unwired: 7 in]
      }
      frame "Test# 9 - OCV final" {
        w360 = 0 ("indice désactivé (ligne)")
        w383 = "0" ("cas faux")
        w384 = "1"
        # "29/08/2022_09:32:18;Test# 3 - BAT+ ;  R = 9999 MOhm;"
        n102 = Index Array(array=w376) -> (element #3=w366:string)  [unwired: 3 in, 2 out]
        n103 = String Subset(string=w366, offset (0)=9) -> (substring=w365:string)  [unwired: 1 in]
        n104 = Increment(x=w372) -> (x+1=w371:i32)
        n105 = Fract/Exp String To Number(string=w365) -> (number=w367:dbl)  [unwired: 3 in, 1 out]
        n106 = In Range and Coerce(upper limit=w353, x=w367, lower limit=w354) -> (In Range?=w364:bool)  [unwired: 1 out]
        n107 = Number To Decimal String(number=w371) -> (decimal integer string=w379:string)  [unwired: 1 in]
        n108 = Select(t=w384, s=w364, f=w383) -> (s? t:f=w382:string)
        n109 = Select(t=w383, s=w364, f=w384) -> (s? t:f=w385:string)
        n110 = call "PASSFAIL.vi"("E"=w364) -> ("S"=w362:string)  [unwired: 10 in]
        n111 = Number To Fractional String(number=w353, precision (6)=i16 3) -> (F-format string=w357:string)  [unwired: 2 in]
        n112 = Number To Fractional String(number=w354, precision (6)=i16 3) -> (F-format string=w358:string)  [unwired: 2 in]
        n113 = Build Array(w379, "OCV final" ("élément"), w382, w385, "NA" ("élément")) -> (w386:string[])
        n114 = call "HTML_Table_Head.vi"("entrée d'erreur (pas d'erreur)"=w375, "Tableau"=w386, "chaîne en entrée"=w373) -> ("sortie d'erreur"=w381:errorcluster, "result string"=w380:string)  [unwired: 7 in]
        n115 = Replace Array Subset(array=string[][] [["Vfinale", "-", "", "", "", "OCV final"]] ("Tableau"), new element #1=w365, index (row) #1=w360, index (col) #1=1 ("indice désactivé (col)"), new element #2=w358, index (row) #2=w360, index (col) #2=2 ("disabled index (col)"), new element #3=w357, index (row) #3=w360, index (col) #3=3 ("disabled index (col)"), new element #4=w362, index (row) #4=w360, index (col) #4=4 ("disabled index (col)")) -> (w369:string[][])
        n116 = call "HTML_Table_Data.vi"("entrée d'erreur (pas d'erreur)"=w381, "Tableau"=w369, "chaîne en entrée"=w380) -> ("sortie d'erreur"=w374:errorcluster, "result string"=w370:string)  [unwired: 7 in]
      }
      frame "NULL", Default {
        # "NULL"
      }
    }
  }
  n117 = call "Recuperation de donnees.vi"("Est-ce un string?"=FALSE, "Array in"=string[][] [["DATA_PARK", "UCELLMAX_MAX"], ["DATA_PARK", "UCELLMAX_MIN"], ["DATA_PARK", "UCELLMIN_MAX"], ["DATA_PARK", "UCELLMIN_MIN"], ["DATA_PARK", "TEMPMAX_MAX"], ["DATA_PARK", "TEMPMAX_MIN"], ["DATA_PARK", "TEMPMIN_MAX"], ["DATA_PARK", "TEMPMIN_MIN"], ["DATA_PARK", "SOH_MAX"], ["DATA_PARK", "SOH_MIN"], ["DATA_PARK", "SOC_MAX"], ["DATA_PARK", "SOC_MIN"], ["DATA_PARK", "VBATT_MAX"], ["DATA_PARK", "VBATT_MIN"], ["DATA_PARK", "IBATT_MAX"], ["DATA_PARK", "IBATT_MIN"]], "Refnum in"=w3) -> ("Array"=→"Array 3":dbl[])  [unwired: 7 in, 1 out]
  n118 = Search and Replace String(replace all?=TRUE ("tout remplacer ? (F)"), input string=w71, search string="<td class=\"core1 testpass\">FAIL</td>" ("chaîne recherchée"), replace string="<td class=\"core1 testfail\">FAIL</td>" ("chaîne de remplacement (\"\")"), error in=w69) -> (result string=w55:string, number of replacements=w50:i32, error out=w66:errorcluster)  [unwired: 3 in, 1 out]
  n119 = Search and Replace String(replace all?=TRUE ("tout remplacer ? (F)"), input string=w55, search string="<td class=\"core1 testpass\">PASS</td>" ("chaîne recherchée"), error in=w66) -> (number of replacements=w58:i32, error out=w62:errorcluster)  [unwired: 4 in, 2 out]
  "nombre de remplacements" <- w58
  n120 = Number To Decimal String(number=w58) -> (decimal integer string=w57:string)  [unwired: 1 in]
  n121 = Number To Decimal String(number=w50) -> (decimal integer string=w56:string)  [unwired: 1 in]
  n122 = Search and Replace String(input string=w55, search string="<!--NBTESTOK-->" ("chaîne recherchée"), replace string=w57, error in=w62) -> (result string=w63:string, error out=w61:errorcluster)  [unwired: 4 in, 2 out]
  n123 = Equal To 0?(x=w50) -> (x = 0?=w41:bool)
  n124 = Search and Replace String(input string=w63, search string="<!--NBTESTKO-->" ("chaîne recherchée"), replace string=w56, error in=w61) -> (result string=w44:string, error out=w49:errorcluster)  [unwired: 4 in, 2 out]
  n125 = Search and Replace String(input string=w44, search string="Résultat du test :\t</td><td class=\"resume5\" colspan=\"3\"><div><span style=\"float:left\" id=\"result\"><font color=\"green\"><b>PASS</b>", replace string="Résultat du test :\t</td><td class=\"resume5\" colspan=\"3\"><div><span style=\"float:left\" id=\"result\"><font color=\"red\"><b>FAIL</b>", error in=w49) -> (result string=w45:string, error out=w48:errorcluster)  [unwired: 4 in, 2 out]
  n126 = Select(t=w44, s=w41, f=w45) -> (s? t:f=w46:string)
  "Chaîne" <- w46
  n127 = Not Equal?(x=w36, y=path "") -> (x != y?=w38:bool)
  n128 = Open/Create/Replace File(file path (use dialog)=w72, error in=w48, operation (0:open)=w54) -> (refnum out=w78:refnum<file>, error out=w80:errorcluster)  [unwired: 3 in, 1 out]
  n129 = case shown="True" w38 {
    tunnel: w54 -> [_ w397]
    tunnel: w36 -> [_ w396]
    tunnel: w48 -> [_ w395]
    tunnel: w46 -> [_ w394]
    tunnel: [errorcluster {"status"=FALSE, "code"=0, "source"=""} ("error out") w393] -> w43
    frame False {
    }
    frame True {
      n130 = Open/Create/Replace File(file path (use dialog)=w396, error in=w395, operation (0:open)=w397) -> (refnum out=w398:refnum<file>, error out=w400:errorcluster)  [unwired: 3 in, 1 out]
      n131 = Write to Text File(file (use dialog)=w398, text=w394, error in=w400) -> (refnum out=w399:refnum<file>, error out=w401:errorcluster)  [unwired: 1 in, 1 out]
      n132 = Close File(refnum=w399, error in=w401) -> (error out=w393:errorcluster)  [unwired: 1 out]
    }
  }
  n133 = Write to Text File(file (use dialog)=w78, text=w46, error in=w80) -> (refnum out=w79:refnum<file>, error out=w81:errorcluster)  [unwired: 1 in, 1 out]
  n134 = Close File(refnum=w79, error in=w81) -> (error out=w42:errorcluster)  [unwired: 1 out]
  n135 = Merge Errors(w42, w43) -> (w40:errorcluster)
  "sortie d'erreur" <- w40
  n136 = Compound Arithmetic op=AND ("Opérateur arithmétique")(w41, invert w40) -> (→"tout bon":bool)
